vi "03_EventStructure4.vi"() -> ()   [LabVIEW 2019]
panel:
  in  "Combo Box":string(combo)
  in  "Enum":enum16{""}(ring)
  in  "Tank":dbl(slide) scale=0.0..10.0
  out "Boolean":bool
  in  "Numeric":dbl
  out "Label.Text":string
  in  "Stop":bool
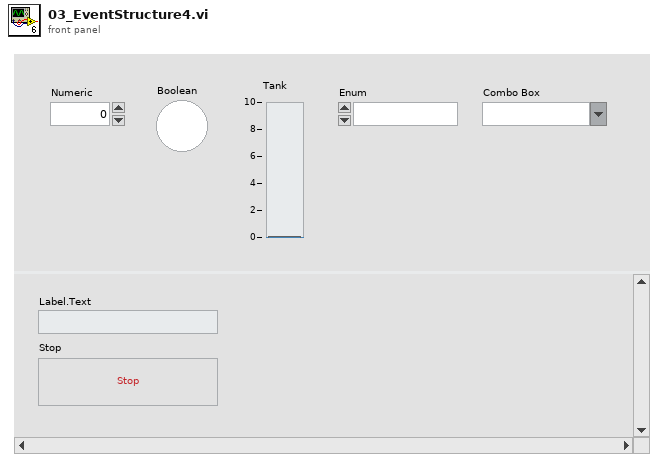
[diagram p1: front panel]
types:
  T1 = typedef "LVPoint32TypeDef.ctl" = cluster{"Horizontal":i32, "Vertical":i32}
  T2 = typedef "LVPositionTypeDef.ctl" = cluster{"Left":i32, "Top":i32}
  T3 = typedef "LVBoundsTypeDef.ctl" = cluster{"Width":u32, "Height":u32}
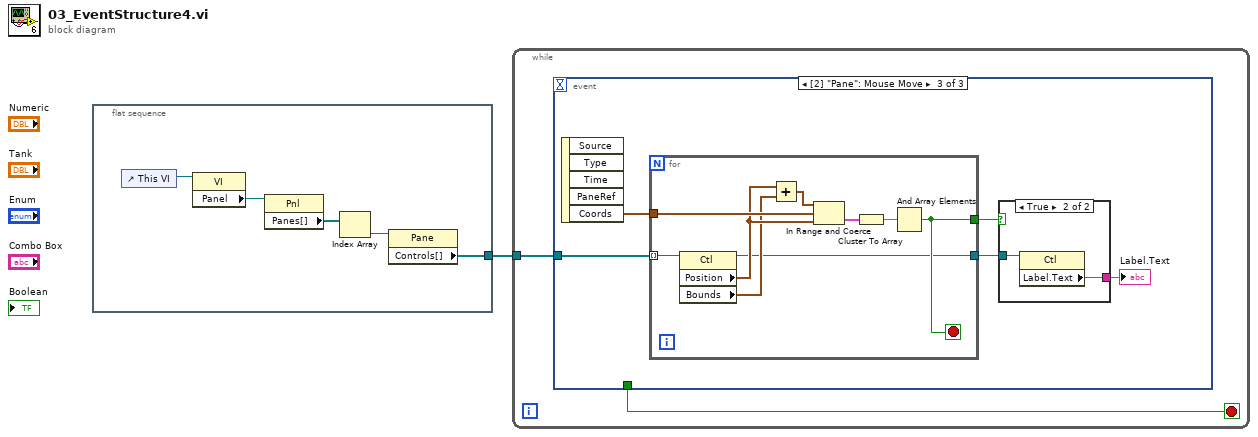
[diagram p0: block diagram]
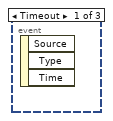
[diagram p2: hidden frame]
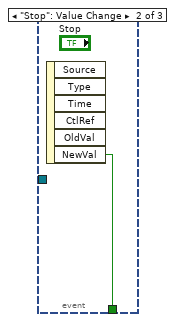
[diagram p3: hidden frame]
diagram:
  n1 = flat-sequence {
    tunnel: [w2] -> w1
    frame #0 {
      n2 = control-ref of="This VI"() -> (w6:refnum<vi>)
      n3 = property class="VI"(reference=w6) -> ("Panel"=w5:refnum<vi>)  [unwired: 1 in, 2 out]
      n4 = property class="Pnl"(reference=w5) -> ("Panes[]"=w4:refnum<vi>[])  [unwired: 1 in, 2 out]
      n5 = Index Array(array=w4) -> (element=w3:refnum<vi>)  [unwired: 1 in]
      n6 = property class="Pane"(reference=w3) -> ("Controls[]"=w2:refnum<vi>[])  [unwired: 1 in, 2 out]
    }
  }
  n7 = while {
    tunnel: w1 -> [w7]
    stop <- w8 stop-if-true
    n8 = event shown="[2] \"Pane\": Mouse Move" {
      selector: _ -> [_ _ _]
      dyn-events: _ -> [_ _ _]
      timeout: _ -> [_ _ _]
      tunnel: [_ w9 _] -> w8
      tunnel: w7 -> [_ _ w14]
      event Timeout {
        n9 = event-data() -> ()  [unwired: 1 in, 3 out]
      }
      event "Stop": Value Change {
        n10 = event-data() -> ("NewVal"=w9:bool)  [unwired: 1 in, 5 out]
      }
      event Mouse Move {
        n11 = event-data() -> ("Coords"=w13:T1)  [unwired: 1 in, 4 out]
        n12 = for {
          tunnel: w14 -> [w25] mode=indexing
          tunnel: w13 -> [w24]
          tunnel: [w18] -> w12
          tunnel: [w17] -> w11
          stop <- w18 stop-if-true
          n13 = property class="Ctl"(reference=w25) -> (reference out=w17:refnum<vi>, "Position"=w23:T2, "Bounds"=w22:T3)  [unwired: 1 in, 1 out]
          n14 = Add(x=w23, y=w22) -> (x+y=w21:T3)
          n15 = In Range and Coerce(upper limit=w21, x=w24, lower limit=w23) -> (In Range?=w20:cluster{"Width":bool, "Height":bool})  [unwired: 1 out]
          n16 = Cluster To Array(cluster=w20) -> (array=w19:bool[])
          n17 = And Array Elements(Boolean array=w19) -> (logical AND=w18:bool)
        }
        n18 = case shown="True" w12 {
          tunnel: w11 -> [_ w16]
          tunnel: [_ w15] -> w10
          frame False {
          }
          frame True {
            n19 = property class="Ctl"(reference=w16) -> ("Label.Text"=w15:string)  [unwired: 1 in, 2 out]
          }
        }
        "Label.Text" <- w10
      }
    }
  }
